vi "Duplicate Service Error.vi"(8 "error in (no error)":errorcluster, 9 "ID":string, 10 "Type":string) -> (0 "error out":errorcluster)   [LabVIEW 2020, in "Vecto.lvlib" / "Service Container.lvclass"]
uses:
  Service Container.lvclass
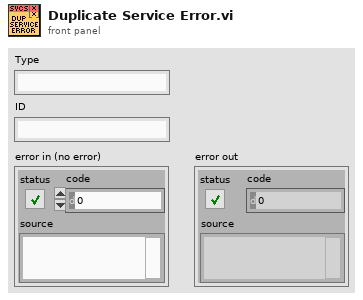
[diagram p1: front panel]
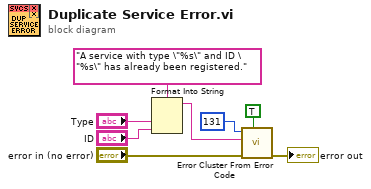
[diagram p0: block diagram]
diagram:
  n1 = Format Into String(format string="A service with type \"%s\" and ID \"%s\" has already been registered.", "Type", "ID") -> (resulting string=w5:string)  [unwired: 2 in, 1 out]
  n2 = call <vilib>:"Error Cluster From Error Code.vi"("show call chain? (False)"=TRUE, "error in (no error)"="error in (no error)", "error message (\"\")"=w5, "error code (0)"=131) -> ("error out"=→"error out":errorcluster)  [unwired: 5 in]
